vi "SaveResultFile.vi"(6 "EN Mark (T)":bool=TRUE, 8 "Fixture_Data":u16[](array[numeric]), 10 "OPC_Model Type":u16 format="%x", 11 "Path":path=path "D:/Output") -> (0 "MarkNG":bool, 2 "FileOutPath":path, 3 "FolderOutPath":path)   [LabVIEW 2017]
uses:
  <vilib>/Utility/file.llb/Write Delimited Spreadsheet (string).vi
panel:
  out "Count":i32
  # "DX = 4458\nK3 = 4B33\n4U = 3455\nWS = 5753\nL5 = 4C53\nKB = 4B42"
  # "00 Product Number"
  # "10 Lane Number"
  # "20 Laser Number"
  # "21 Laser Number"
  # "30 Fixture Result"
  # "40 Master Unit"
  # "60 Mega Test"
  # "70 Windows Lock Press"
  # "71 Windows Lock Unpress"
  # "80 Door Lock"
  # "81 Door Unlock"
  # "90 FR Man Up"
  # "91 FR Man Down"
  # "92 FR Auto Up"
  # "93 FR Auto Down"
  # "100 RR Man Up"
  # "101 RR Man Down"
  # "110 FL Man Up"
  # "111 FL Man Down"
  # "112 FL Auto Up"
  # "113 FL  Down"
  # "120 RL Man Up"
  # "121 RL Man Down"
  # "130 LIN DR Up Contact"
  # "131 LIN DR Down Contact"
  # "132 LIN DR Auto Status"
  # "133 LIN AS Up Contact"
  # "134 LIN AS Down Contact"
  # "135 LIN AS Auto Status"
  # "136 WDW Lock Status"
  # "140 Vision Illumination"
  # "150 Vision Pin"
  # "160 QR Code Reader"
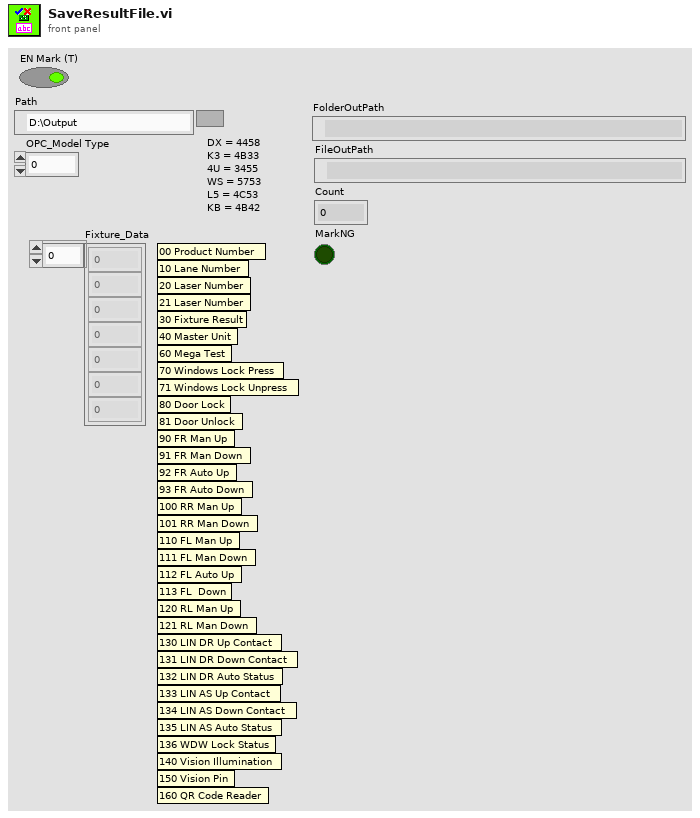
[diagram p1: front panel]
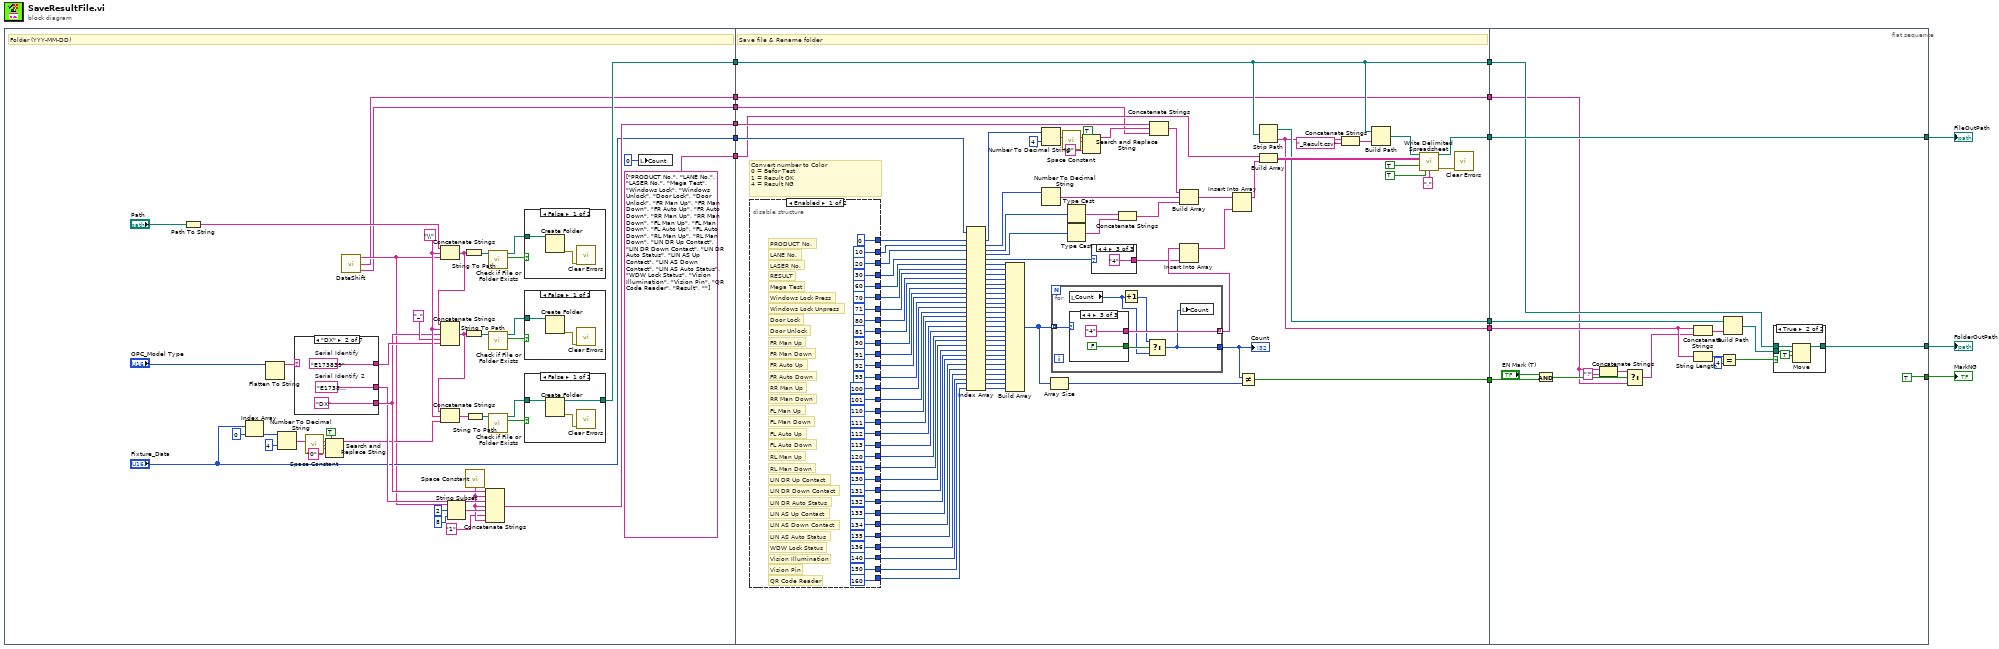
[diagram p0: block diagram]
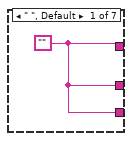
[diagram p4: hidden frame]
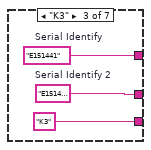
[diagram p5: hidden frame]
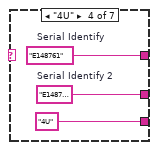
[diagram p6: hidden frame]
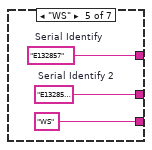
[diagram p7: hidden frame]
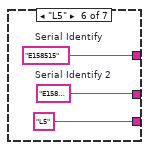
[diagram p8: hidden frame]
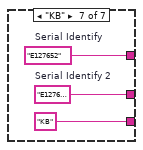
[diagram p9: hidden frame]
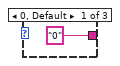
[diagram p11: hidden frame]
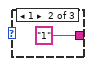
[diagram p12: hidden frame]
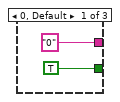
[diagram p13: hidden frame]
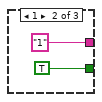
[diagram p14: hidden frame]
diagram:
  n1 = flat-sequence {
    tunnel: [w37] -> w7
    tunnel: [string[] ["PRODUCT No.", "LANE No.", "LASER No.", "Mega Test", "Windows Lock", "Windows Unlock", "Door Lock", "Door Unlock", "FR Man Up", "FR Man Down", "FR Auto Up", "FR Auto Down", "RR Man Up", "RR Man Down", "FL Man Up", "FL Man Down", "FL Auto Up", "FL Auto Down", "RL Man Up", "RL Man Down", "LIN DR Up Contact", "LIN DR Down Contact", "LIN DR Auto Status", "LIN AS Up Contact", "LIN AS Down Contact", "LIN AS Auto Status", "WDW Lock Status", "Vision Illumination", "Vision Pin", "QR Code Reader", "Result", ""]] -> w6
    tunnel: ["Fixture_Data"] -> w5
    tunnel: [w31] -> w4
    tunnel: [w17] -> w3
    tunnel: [w16] -> w1
    tunnel: [w176] -> w15
    tunnel: [w175] -> w14
    tunnel: [w174] -> w13
    tunnel: [w173] -> w12
    tunnel: [w172] -> w11
    tunnel: w7 -> [w173]
    tunnel: w6 -> [w96]
    tunnel: w5 -> [w116]
    tunnel: w4 -> [w110]
    tunnel: w3 -> [w86]
    tunnel: [w85] -> w2
    tunnel: w1 -> [w85]
    tunnel: [w248] -> w10
    tunnel: w15 -> [w248]
    tunnel: w14 -> [w246]
    tunnel: w13 -> [w245]
    tunnel: w12 -> [w244]
    tunnel: w11 -> [w243]
    tunnel: [w242] -> w9
    tunnel: [TRUE] -> w8
    tunnel: w2 -> [w233]
    frame #0 {
      w40 = "\\" ("string")
      # "Folder (YYY-MM-DD)"
      n2 = Path To String(path="Path") -> (string=w53:string)
      n3 = Index Array(array="Fixture_Data", index=0) -> (element=w25:u16)
      n4 = Flatten To String(anything="OPC_Model Type") -> (data string=w49:string)  [unwired: 3 in, 2 out]
      n5 = Number To Decimal String(number=w25, width (-)=i16 4) -> (decimal integer string=w24:string)
      n6 = case shown="\"DX\"" w49 {
        tunnel: [w64 w67 w70 w73 w76 w79 w82] -> w36
        tunnel: [w64 "DX" "K3" "4U" "WS" "L5" "KB"] -> w35
        tunnel: [w64 w65 w68 w71 w74 w77 w80] -> w34
        frame " ", Default {
          w64 = ""
        }
        frame "DX" {
          w65 = "E173839 254016PA3A"  # Serial Identify 2
          w67 = "E173839"  # Serial Identify
        }
        frame "K3" {
          w68 = "E151441 254016PA2A"  # Serial Identify 2
          w70 = "E151441"  # Serial Identify
        }
        frame "4U" {
          w71 = "E148761 254016PA1A"  # Serial Identify 2
          w73 = "E148761"  # Serial Identify
        }
        frame "WS" {
          w74 = "E132857 254016LA1A"  # Serial Identify 2
          w76 = "E132857"  # Serial Identify
        }
        frame "L5" {
          w77 = "E158515 254016LA2A"  # Serial Identify 2
          w79 = "E158515"  # Serial Identify
        }
        frame "KB" {
          w80 = "E127652 254016LA0A"  # Serial Identify 2
          w82 = "E127652"  # Serial Identify
        }
      }
      n7 = call <vilib>:"Space Constant.vi"() -> ("String"=w29:string)
      n8 = Search and Replace String(replace all?=TRUE ("replace all? (F)"), input string=w24, search string=w29, replace string="0" ("replace string (\"\")")) -> (result string=w21:string)  [unwired: 4 in, 3 out]
      n9 = call "DateShift.vi"() -> ("RealTime"=w17:string, "NameTime"=w16:string, "DateShift"=w18:string)  [unwired: 3 in]
      n10 = Concatenate Strings(w53, w40, w18) -> (w45:string)
      n11 = Concatenate Strings(w45, w40, w35, "_" ("string"), w36) -> (w39:string)
      n12 = Concatenate Strings(w39, w40, w21) -> (w44:string)
      n13 = String Subset(string=w18, offset (0)=2, length (rest)=8 ("length (rest)")) -> (substring=w32:string)
      n14 = String To Path(string=w45) -> (path=w54:path)
      n15 = String To Path(string=w39) -> (path=w48:path)
      n16 = String To Path(string=w44) -> (path=w41:path)
      n17 = call <vilib>:"Space Constant.vi"() -> ("String"=w30:string)
      n18 = Concatenate Strings(w35, w30, w34, w30, w32, "1" ("string"), w30) -> (w31:string)
      n19 = call <vilib>:"Check if File or Folder Exists.vi"("path"=w54) -> ("file or folder exists?"=w55:bool, "dup path"=w56:path)  [unwired: 8 in, 1 out]
      n20 = call <vilib>:"Check if File or Folder Exists.vi"("path"=w48) -> ("file or folder exists?"=w47:bool, "dup path"=w46:path)  [unwired: 8 in, 1 out]
      n21 = call <vilib>:"Check if File or Folder Exists.vi"("path"=w41) -> ("file or folder exists?"=w42:bool, "dup path"=w43:path)  [unwired: 8 in, 1 out]
      n22 = case shown="False" w55 {
        tunnel: w56 -> [w84 _]
        frame False {
          n23 = Create Folder(path (use dialog)=w84) -> (error out=w83:errorcluster)  [unwired: 2 in, 2 out]
          n24 = call <vilib>:"Clear Errors.vi"("error in (no error)"=w83) -> ()  [unwired: 5 in, 2 out]
        }
        frame True {
        }
      }
      n25 = case shown="False" w47 {
        tunnel: w46 -> [w63 _]
        frame False {
          n26 = Create Folder(path (use dialog)=w63) -> (error out=w62:errorcluster)  [unwired: 2 in, 2 out]
          n27 = call <vilib>:"Clear Errors.vi"("error in (no error)"=w62) -> ()  [unwired: 5 in, 2 out]
        }
        frame True {
        }
      }
      n28 = case shown="False" w42 {
        tunnel: w43 -> [w60 w61]
        tunnel: [w58 w61] -> w37
        frame False {
          n29 = Create Folder(path (use dialog)=w60) -> (created path=w58:path, error out=w59:errorcluster)  [unwired: 2 in, 1 out]
          n30 = call <vilib>:"Clear Errors.vi"("error in (no error)"=w59) -> ()  [unwired: 5 in, 2 out]
        }
        frame True {
        }
      }
      n31 = local write "Count"(0 ("Count")) -> ()
    }
    frame #1 {
      # "Convert number to Color\n0 = Befor Test\n1 = Result OK\n4 = Result NG"
      # "Save file & Rename folder"
      n32 = disable-structure shown="Enabled" {
        disable-tunnel: [60 ("index") _] -> w109
        disable-tunnel: [70 ("index") _] -> w171
        disable-tunnel: [71 ("index") _] -> w170
        disable-tunnel: [80 ("index") _] -> w169
        disable-tunnel: [81 ("index") _] -> w168
        disable-tunnel: [90 ("index") _] -> w167
        disable-tunnel: [91 ("index") _] -> w166
        disable-tunnel: [92 ("index") _] -> w165
        disable-tunnel: [93 ("index") _] -> w164
        disable-tunnel: [100 ("index") _] -> w163
        disable-tunnel: [101 ("index") _] -> w162
        disable-tunnel: [110 ("index") _] -> w161
        disable-tunnel: [111 ("index") _] -> w160
        disable-tunnel: [112 ("index") _] -> w159
        disable-tunnel: [113 ("index") _] -> w158
        disable-tunnel: [120 ("index") _] -> w157
        disable-tunnel: [121 ("index") _] -> w156
        disable-tunnel: [130 ("index") _] -> w155
        disable-tunnel: [131 ("index") _] -> w154
        disable-tunnel: [132 ("index") _] -> w153
        disable-tunnel: [133 ("index") _] -> w152
        disable-tunnel: [134 ("index") _] -> w151
        disable-tunnel: [135 ("index") _] -> w150
        disable-tunnel: [136 ("index") _] -> w149
        disable-tunnel: [140 ("index") _] -> w148
        disable-tunnel: [150 ("index") _] -> w147
        disable-tunnel: [160 ("index") _] -> w146
        disable-tunnel: [0 ("index") _] -> w108
        disable-tunnel: [10 ("index") _] -> w105
        disable-tunnel: [20 ("index") _] -> w104
        disable-tunnel: [30 ("index") _] -> w103
        frame Enabled {
          # "LASER No."
          # "RESULT"
          # "LANE No."
          # "PRODUCT No."
          # "WDW Lock Status"
          # "QR Code Reader"
          # "Vision Pin"
          # "Vision Illumination"
          # "LIN AS Auto Status"
          # "LIN AS Down Contact"
          # "LIN AS Up Contact"
          # "LIN DR Auto Status"
          # "LIN DR Down Contact"
          # "LIN DR Up Contact"
          # "RL Man Down"
          # "RL Man Up"
          # "FL Auto Down"
          # "FL Auto Up"
          # "FL Man Down"
          # "FL Man Up"
          # "RR Man Down"
          # "RR Man Up"
          # "FR Auto Down"
          # "FR Auto Up"
          # "FR Man Down"
          # "FR Man Up"
          # "Door Unlock"
          # "Door Lock"
          # "Windows Lock Unpress"
          # "Windows Lock Press"
          # "Mega Test"
        }
        frame Disabled {
        }
      }
      n33 = Index Array(array=w116, index #1=w108, index #2=w105, index #3=w104, index #5=w103, index #6=w109, index #7=w171, index #8=w170, index #9=w169, index #10=w168, index #11=w167, index #12=w166, index #13=w165, index #14=w164, index #15=w163, index #16=w162, index #17=w161, index #18=w160, index #19=w159, index #20=w158, index #21=w157, index #22=w156, index #23=w155, index #24=w154, index #25=w153, index #26=w152, index #27=w151, index #28=w150, index #29=w149, index #30=w148, index #31=w147, index #32=w146) -> (element #1=w90:u16, element #2=w88:u16, element #3=w107:u16, element #4=w106:u16, element #5=w101:u16, element #6=w102:u16, element #7=w145:u16, element #8=w144:u16, element #9=w143:u16, element #10=w142:u16, element #11=w141:u16, element #12=w140:u16, element #13=w139:u16, element #14=w138:u16, element #15=w137:u16, element #16=w136:u16, element #17=w135:u16, element #18=w134:u16, element #19=w133:u16, element #20=w132:u16, element #21=w131:u16, element #22=w130:u16, element #23=w129:u16, element #24=w128:u16, element #25=w127:u16, element #26=w126:u16, element #27=w125:u16, element #28=w124:u16, element #29=w123:u16, element #30=w122:u16, element #31=w121:u16, element #32=w120:u16)  [unwired: 1 in]
      n34 = Build Array(w102, w145, w144, w143, w142, w141, w140, w139, w138, w137, w136, w135, w134, w133, w132, w131, w130, w129, w128, w127, w126, w125, w124, w123, w122, w121, w120) -> (w119:u16[])
      n35 = Number To Decimal String(number=w90, width (-)=i16 4) -> (decimal integer string=w92:string)
      n36 = Number To Decimal String(number=w88) -> (decimal integer string=w87:string)  [unwired: 1 in]
      n37 = Array Size(array=w119) -> (size(s)=w117:i32)
      n38 = for {
        tunnel: w119 -> [w193] mode=indexing
        tunnel: [w192] -> w99 mode=indexing
        tunnel: [w188] -> w118
        n39 = local read "Count"() -> (w189:i32)
        n40 = case shown="4" w193 {
          tunnel: ["0" "1" "4"] -> w192
          tunnel: [TRUE TRUE FALSE] -> w191
          frame 0, Default {
          }
          frame 1 {
          }
          frame 4 {
          }
        }
        n41 = Increment(x=w189) -> (x+1=w190:i32)
        n42 = Select(t=w190, s=w191, f=w189) -> (s? t:f=w188:i32)
        n43 = local write "Count"(w188) -> ()
      }
      "Count" <- w118
      n44 = call <vilib>:"Space Constant.vi"() -> ("String"=w95:string)
      n45 = Type Cast(x=w107) -> (*(type *) &x=w114:string)  [unwired: 1 in]
      n46 = Type Cast(x=w106) -> (*(type *) &x=w115:string)  [unwired: 1 in]
      n47 = Search and Replace String(replace all?=TRUE ("replace all? (F)"), input string=w92, search string=w95, replace string="0" ("replace string (\"\")")) -> (result string=w89:string)  [unwired: 4 in, 3 out]
      n48 = case shown="4" w101 {
        tunnel: ["0" "1" "4"] -> w98
        frame 0, Default {
        }
        frame 1 {
        }
        frame 4 {
        }
      }
      n49 = Concatenate Strings(w114, w115) -> (w113:string)
      n50 = Concatenate Strings(w110, w89, w86) -> (w111:string)
      n51 = Build Array(w111, w87, w113) -> (w97:string[])
      n52 = Insert Into Array(array=w99, new element=w98) -> (w100:string[])  [unwired: 1 in]
      n53 = Insert Into Array(array=w97, new element=w100) -> (w112:string[])  [unwired: 1 in]
      n54 = Not Equal?(x=w118, y=w117) -> (x != y?=w172:bool)
      n55 = Strip Path(path=w173) -> (stripped path=w175:path, name=w174:string)
      n56 = Build Array(w96, w112) -> (w177:string[][])
      n57 = Concatenate Strings(w174, "_Result.csv" ("string")) -> (w183:string)
      n58 = Build Path(base path=w173, name or relative path=w183) -> (appended path=w184:path)
      n59 = call-poly <vilib>:"Write Delimited Spreadsheet.vi"("file path (dialog if empty)"=w184, "2D data"=w177, "append to file? (new file:F)"=TRUE, "transpose? (no:F)"=TRUE, "delimiter (\\t)"="," ("delimiter (\\t)")) -> ("new file path (Not A Path if cancelled)"=w176:path, "error out"=w182:errorcluster)  [unwired: 9 in]
      n60 = call <vilib>:"Clear Errors.vi"("error in (no error)"=w182) -> ()  [unwired: 5 in, 2 out]
    }
    frame #2 {
      n61 = And(x="EN Mark (T)", y=w243) -> (x .and. y?=w235:bool)
      n62 = Concatenate Strings(w233, "!" ("string")) -> (w232:string)
      n63 = Select(t=w232, s=w235, f=w233) -> (s? t:f=w234:string)
      n64 = Concatenate Strings(w245, w234) -> (w237:string)
      n65 = String Length(string=w245) -> (length=w240:i32)
      n66 = Equal?(x=w240, y=4) -> (x = y?=w238:bool)
      n67 = Build Path(base path=w246, name or relative path=w237) -> (appended path=w236:path)
      n68 = case shown="True" w238 {
        tunnel: w244 -> [w249 w253]
        tunnel: [w249 w252] -> w242
        tunnel: w236 -> [_ w250]
        frame False {
        }
        frame True {
          n69 = Move(source path=w253, 9:TRUE ("overwrite (F)"), 10:w250) -> (3:w252:path)  [unwired: 2 in, 2 out]
        }
      }
    }
  }
  "FolderOutPath" <- w9
  "MarkNG" <- w8
  "FileOutPath" <- w10
